vi "英维克空调.vi"() -> ()   [LabVIEW 2016, in "环境动力监测库.lvlib" / "空调库.lvlib"]
panel:
  out "x+1":u32
  in  "解除告警":bool
  out "串口":string
  in  "查看型号":bool
  out "遥控开关机状态":bool
  in  "重开串口":bool
  in  "设定参数":bool
  in  "遥控":bool
  out "系统参数":T1
  out "告警状态":T2
  out "传感器状态":T3
  out "运行状态":T4
  out "通讯":bool
  # "℃"
  # "℃"
  # "℃"
  # "℃"
  # "℃"
  # "℃"
  # "%"
  # "℃"
  # "℃"
  # "℃"
  # "℃"
  # "℃"
  # "%"
  # "℃"
  # "A"
  # "V"
  # "V"
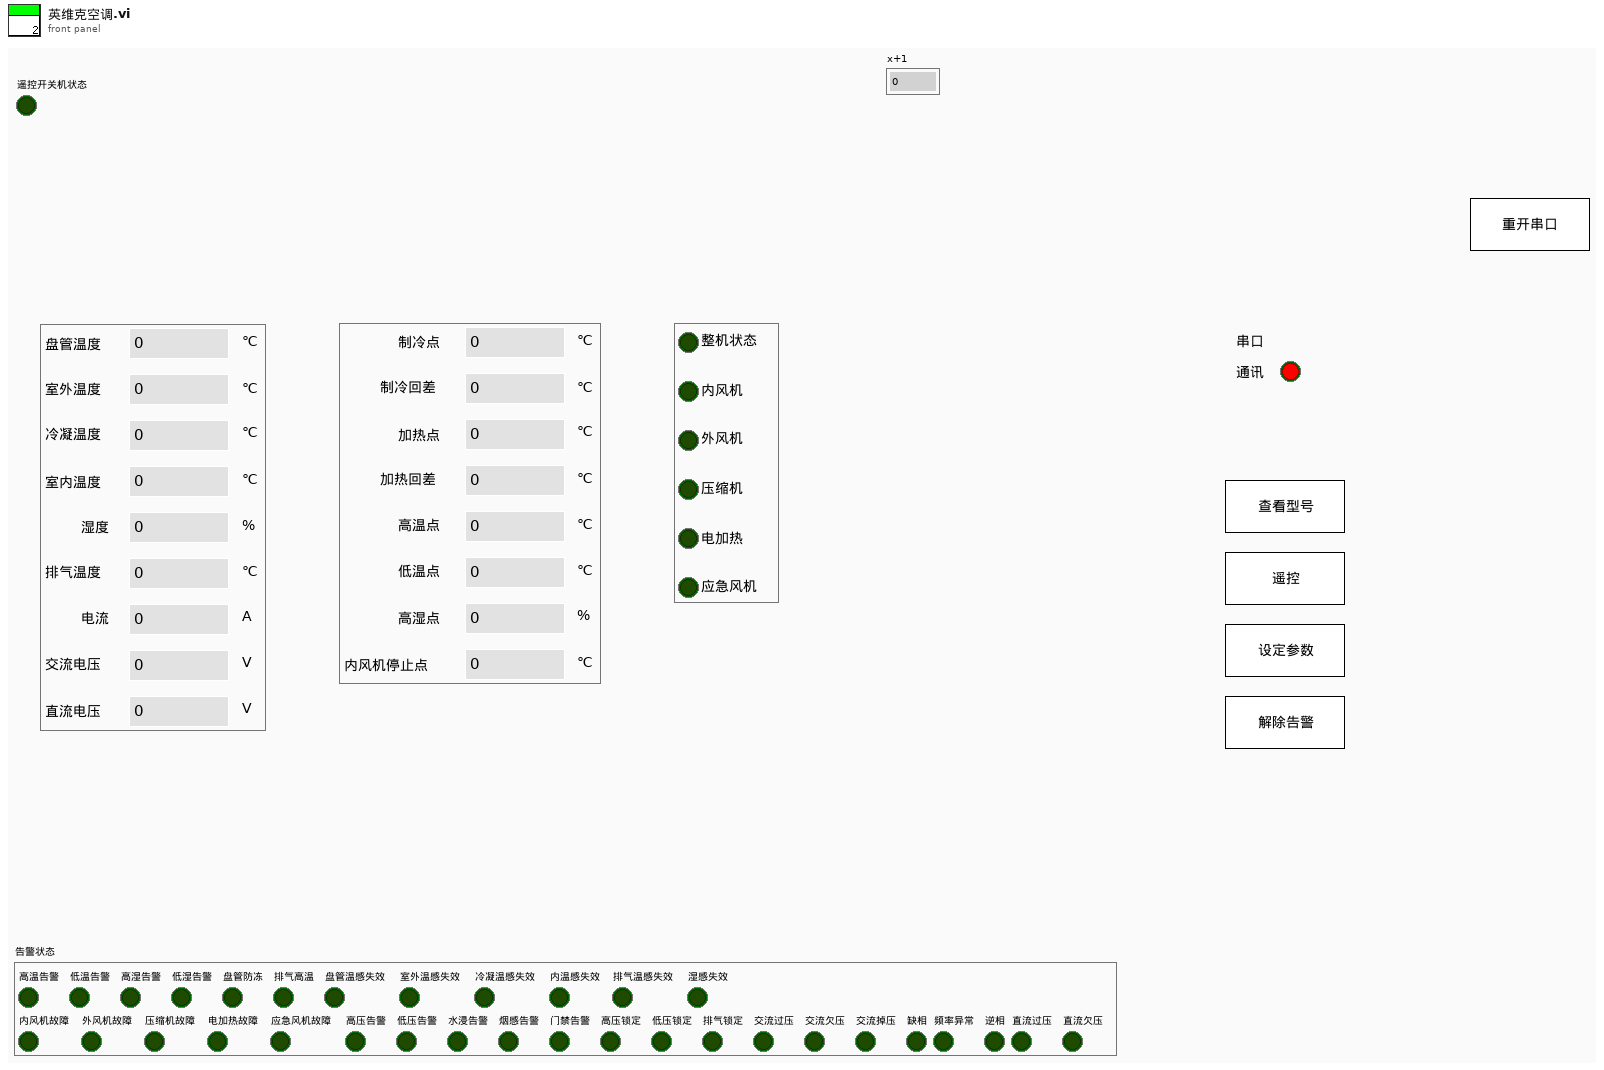
[diagram p1: front panel]
types:
  T1 = cluster{"制冷点":u16, "制冷回差":u16, "加热点":u16, "加热回差":u16, "预留":u16, "预留":u16, "高温点":u16, "低温点":u16, "高湿点":u16, "内风机停止点":u16}
  T2 = cluster{"高温告警":bool, "低温告警":bool, "高湿告警":bool, "低湿告警":bool, "盘管防冻":bool, "排气高温":bool, "盘管温感失效":bool, "室外温感失效":bool, "冷凝温感失效":bool, "内温感失效":bool, "排气温感失效":bool, "湿感失效":bool, "内风机故障":bool, "外风机故障":bool, "压缩机故障":bool, "电加热故障":bool, "应急风机故障":bool, "高压告警":bool, "低压告警":bool, "水浸告警":bool, "烟感告警":bool, "门禁告警":bool, "高压锁定":bool, "低压锁定":bool, "排气锁定":bool, "交流过压":bool, "交流欠压":bool, "交流掉压":bool, "缺相":bool, "频率异常":bool, "逆相":bool, "直流过压":bool, "直流欠压":bool}
  T3 = cluster{"盘管温度":u16, "室外温度":u16, "冷凝温度":u16, "室内温度":u16, "湿度":u16, "排气温度":u16, "电流":u16, "交流电压":u16, "直流电压":u16}
  T4 = cluster{"整机状态":bool, "内风机":bool, "外风机":bool, "压缩机":bool, "电加热":bool, "应急风机":bool}
  T5 = cluster{"型号选择":enum16{"黑盾", "英维克", "仁科测控RS-KTC-N01"}, "MB session in":refnum<class "MB_Master.lvclass">, "英维克空调寄存器":u16[], "通讯状态":bool, "PORT":string, "IP":string, "Slave ID ":u8, "Serial Config":cluster{"baud rate (bps)":u32, "stop bits":u16, "parity":u16, "flow control":u16, "timeout":u32, "retries":i32}, "VISA Resource":refnum<visa-resource-name>, "MB通信方式选择":enum16{"串口", "TCP"}, "系统参数":cluster{"空调开启点":u16, "空调灵敏点":u16, "加热开启点":u16, "加热灵敏度":u16, "高温告警点":u16, "低温告警点":u16}}
  T6 = cluster{"制冷点":u16, "制冷回差":u16, "加热点":u16, "加热回差":u16, "保留":u16, "保留":u16, "高温点":u16, "低温点":u16, "高湿点":u16, "内风机停止点":u16}
  T7 = cluster{"温湿度":cluster{"状态":bool, "温度:":sgl, "湿度:":sgl, "详情  ":bool}, "空调":cluster{"状态":bool, "机柜温度:":sgl, "压缩机:":enum16{"停止", "运行"}, "电加热:":enum16{"停止", "运行"}, "详情  ":bool}, "排气扇":cluster{"排气扇":bool, "详情  ":bool}, "冰箱":cluster{"冰箱":bool, "详情  ":bool}}
  T8 = enum16{"open", "read", "write single", "write", "close"}
  T9 = enum16{"空调制冷点", "空调制冷回差", "加热点", "加热回差", "高温点", "低温点", "高湿点", "内风机停止点"}
  T10 = cluster{"漏水监测输出":cluster{"漏水监测告警":bool, "告警内容":string}, "门禁监测输出":cluster{"门禁监测告警":bool, "告警内容":string}, "门禁监测输出2":cluster{"门禁监测告警":bool, "告警内容":string}, "温湿度监测输出":cluster{"温湿度监测告警":bool, "告警内容":string}, "烟雾监测输出":cluster{"烟雾监测告警":bool, "告警内容":string}, "空调监测输出":cluster{"空调监测告警":bool, "告警内容":string}, "自动重合闸输出":cluster{"自动重合闸告警":bool, "告警内容":string}, "红外入侵输出":cluster{"红外入侵告警":bool, "告警内容":string}, "振动输出":cluster{"振动告警":bool, "告警内容":string}, "UPS输出":cluster{"UPS告警":bool, "告警内容":string}, "蓄电池输出":cluster{"蓄电池告警":bool, "告警内容":string}, "蓄电池输出2":cluster{"蓄电池告警":bool, "告警内容":string}, "GPS输出":cluster{"定位告警":bool, "告警内容":string}, "北斗输出":cluster{"定位告警":bool, "告警内容":string}, "气象输出":cluster{"气象告警":bool, "告警内容":string}, "废液输出":cluster{"废液告警":bool, "告警内容":string}, "废液输出2":cluster{"废液告警":bool, "告警内容":string}}
  T11 = enum32{"Bad", "Idle", "Run top level", "Running"}
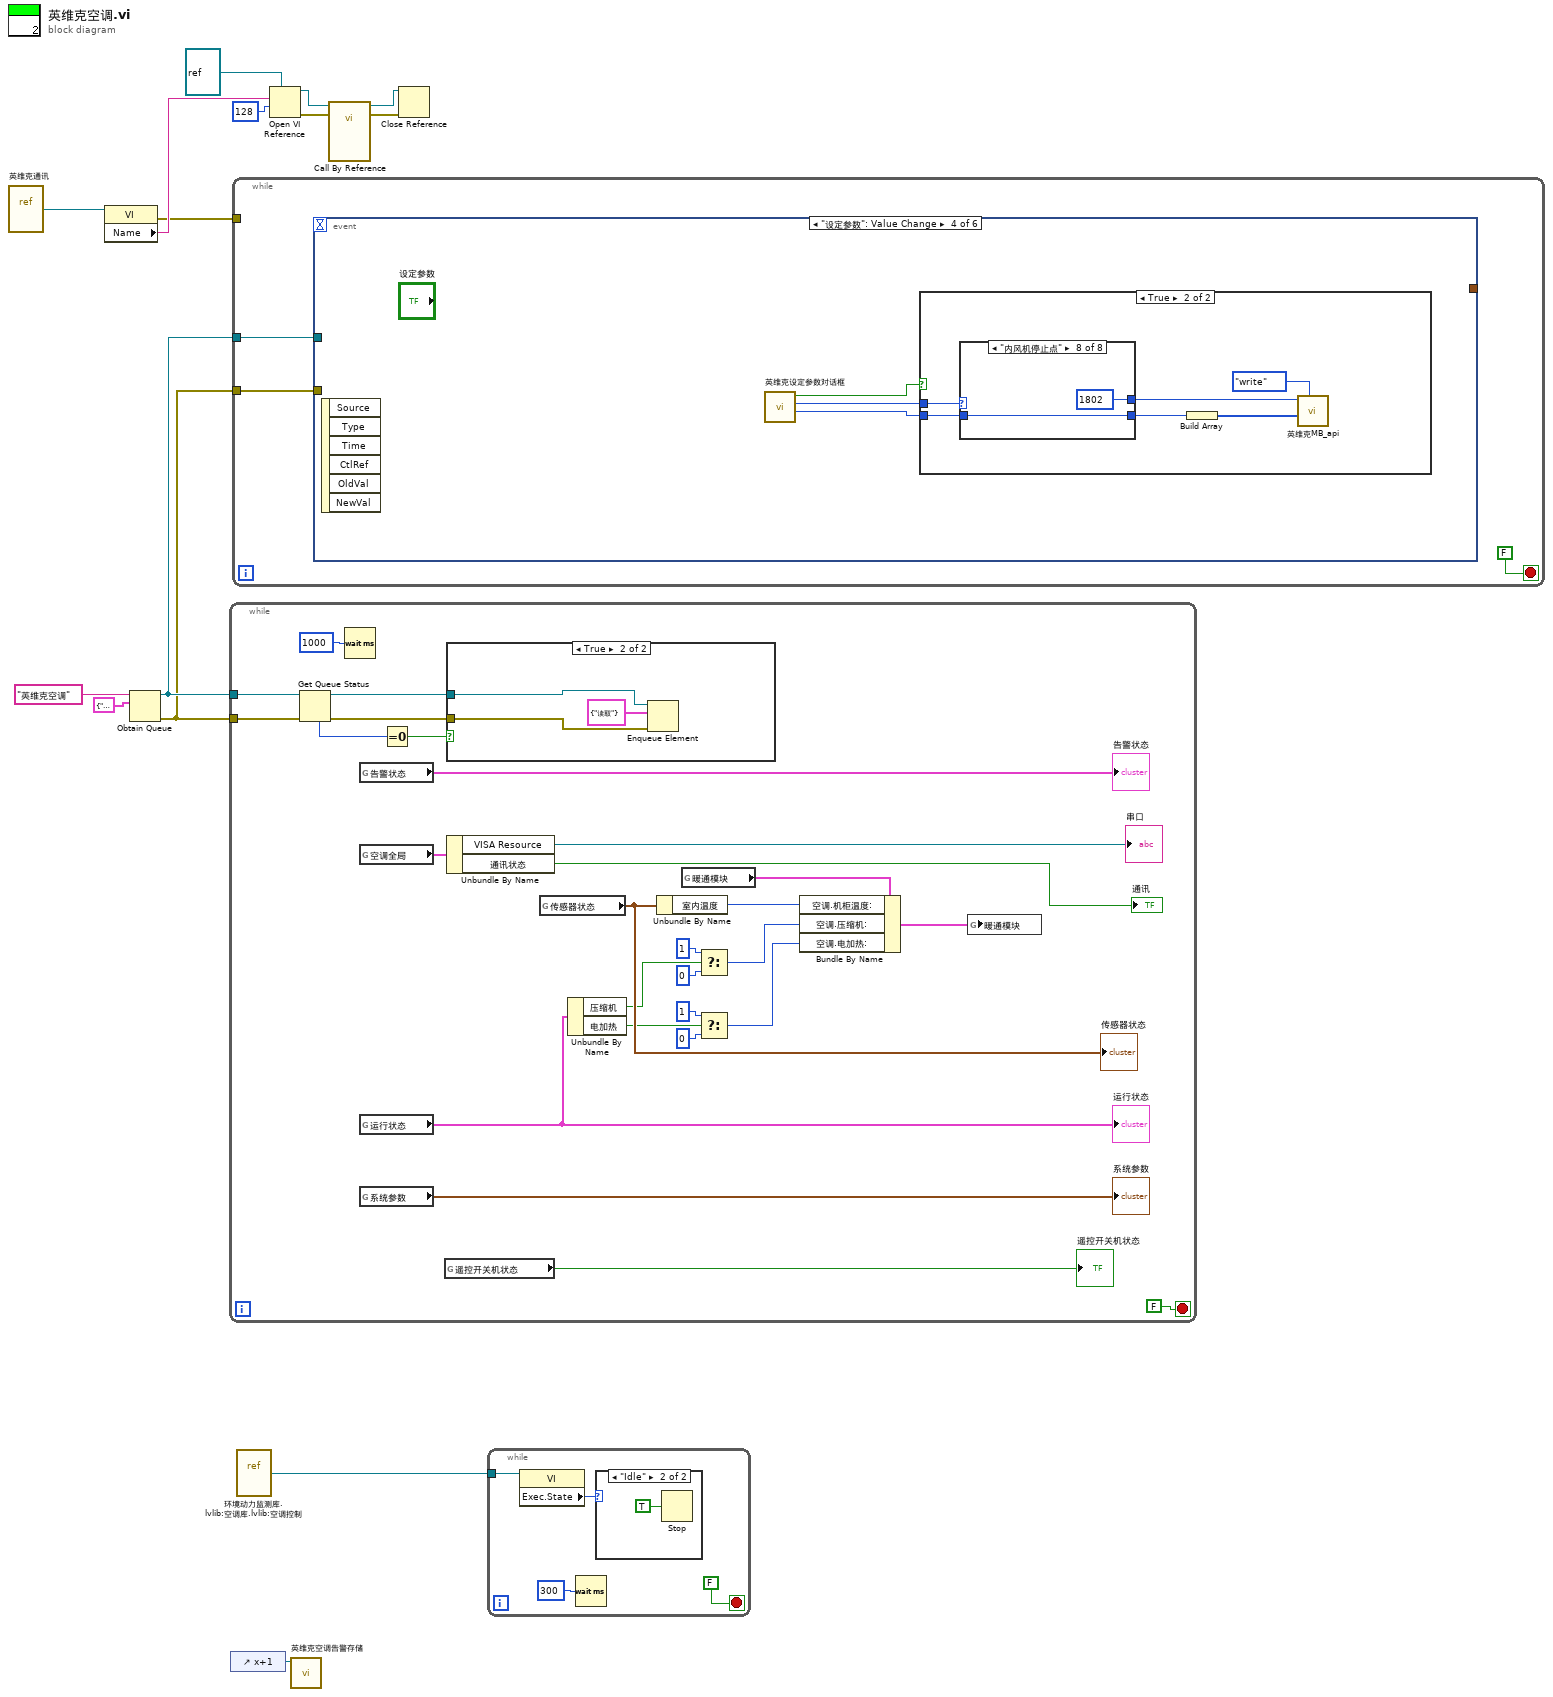
[diagram p0: block diagram]
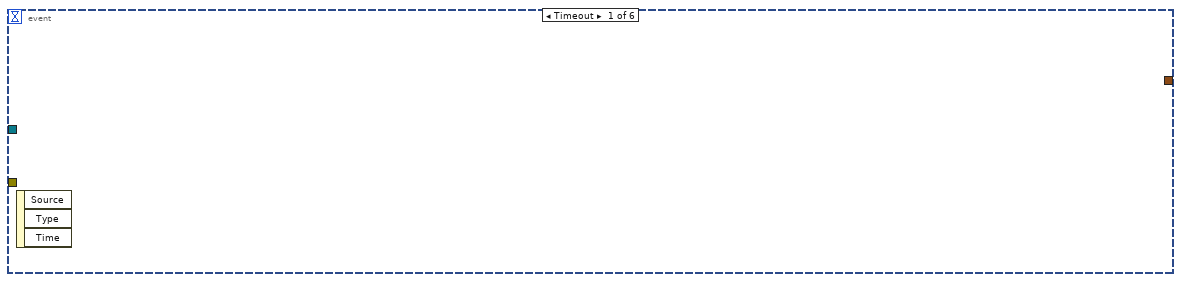
[diagram p4: hidden frame]
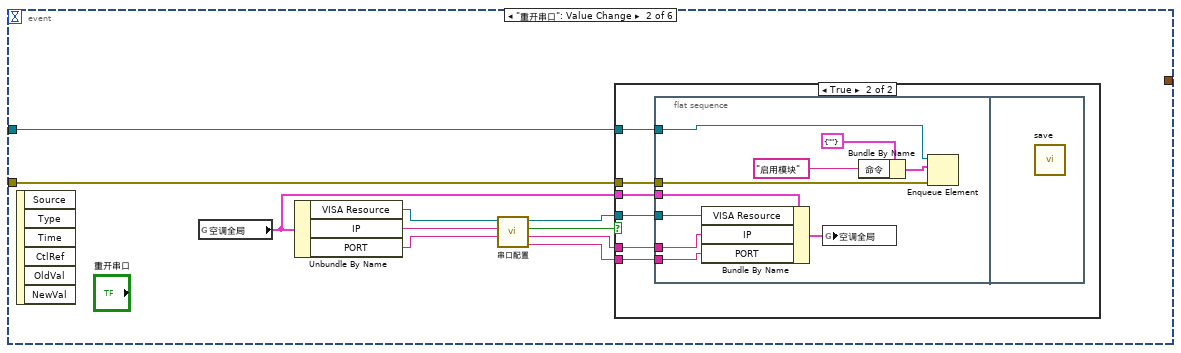
[diagram p5: hidden frame]
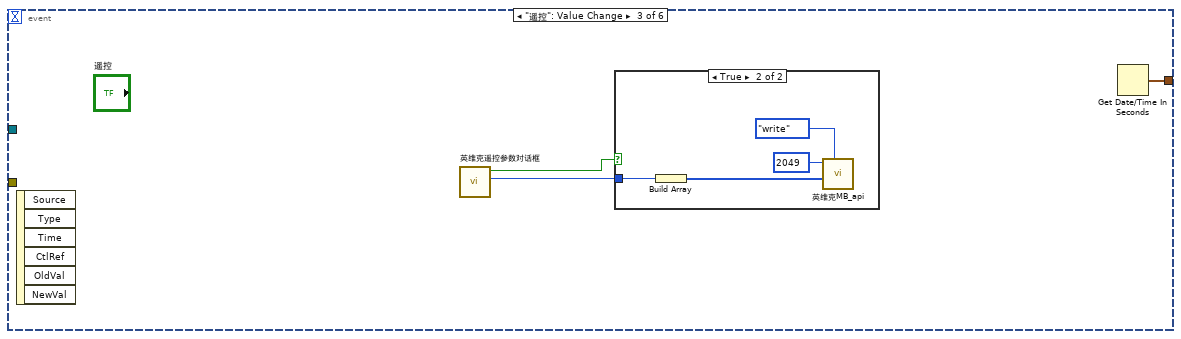
[diagram p7: hidden frame]
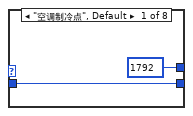
[diagram p10: hidden frame]
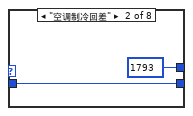
[diagram p11: hidden frame]
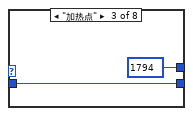
[diagram p12: hidden frame]
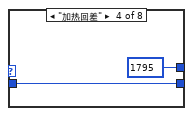
[diagram p13: hidden frame]
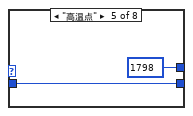
[diagram p14: hidden frame]
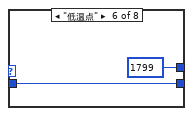
[diagram p15: hidden frame]
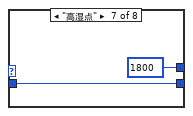
[diagram p16: hidden frame]
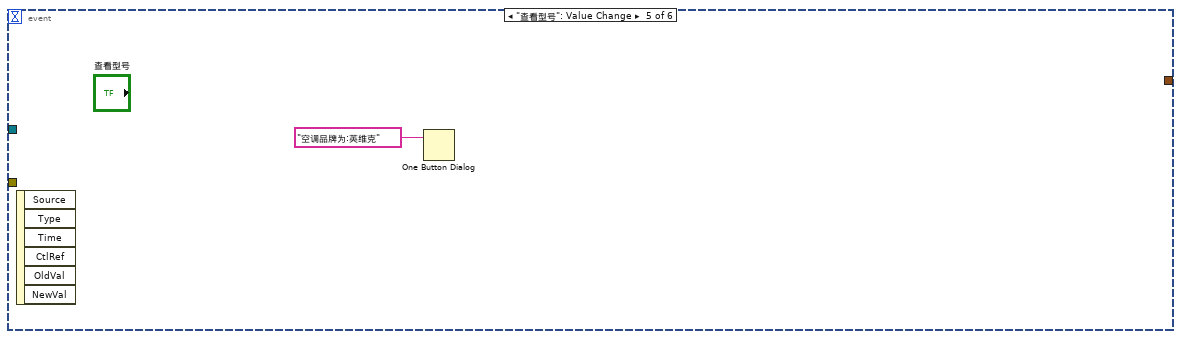
[diagram p17: hidden frame]
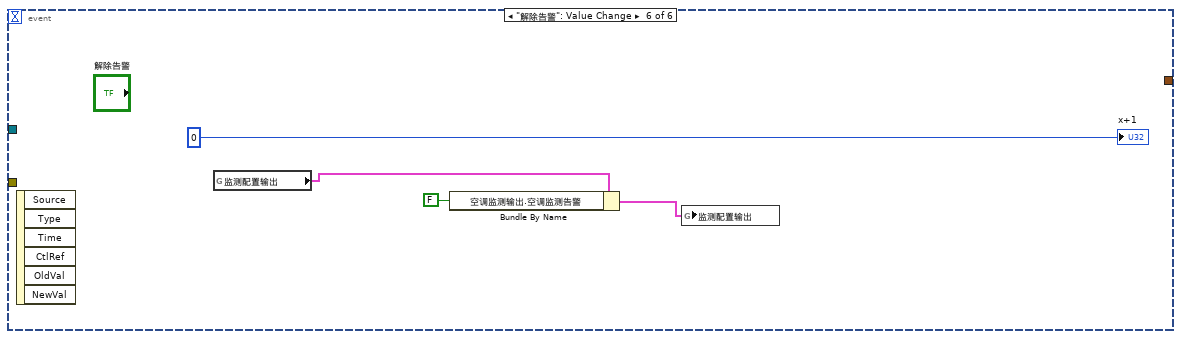
[diagram p18: hidden frame]
diagram:
  n1 = vi-ref "英维克通讯.vi"() -> (w8:refnum<vi>)
  n2 = property class="VI"(reference=w8) -> (error out=w3:errorcluster, "Name"=w9:string)  [unwired: 1 in, 1 out]
  n3 = Obtain Queue(name (unnamed)="英维克空调" ("名称（未命名）"), element data type=cluster{"命令":string} {"命令"="启用模块"} ("元素")) -> (queue out=w5:refnum<queue>, error out=w4:errorcluster)  [unwired: 3 in, 1 out]
  n4 = while {
    tunnel: w5 -> [w41]
    tunnel: w4 -> [w40]
    stop <- FALSE stop-if-true
    n5 = Get Queue Status(queue=w41, error in (no error)=w40) -> (queue out=w38:refnum<queue>, error out=w37:errorcluster, # elements in queue=w42:i32)  [unwired: 1 in, 5 out]
    n6 = Wait (ms)(milliseconds to wait=u32 1000 ("等待时间（毫秒）")) -> ()  [unwired: 1 out]
    n7 = global read "内部交互全局变量.vi" "告警状态"() -> (→"告警状态":T2)
    n8 = global read "断电保存全局变量.vi" "空调全局"() -> (w18:T5)
    n9 = global read "内部交互全局变量.vi" "运行状态"() -> (w27:T4)
    "运行状态" <- w27
    n10 = global read "内部交互全局变量.vi" "系统参数"() -> (→"系统参数":T6)
    n11 = Equal To 0?(x=w42) -> (x = 0?=w39:bool)
    n12 = global read "内部交互全局变量.vi" "遥控开关机状态"() -> (→"遥控开关机状态":bool)
    n13 = case shown="True" w39 {
      tunnel: w38 -> [_ w45]
      tunnel: w37 -> [_ w44]
      frame False {
      }
      frame True {
        n14 = Enqueue Element(queue=w45, element=cluster{"命令":string} {"命令"="读取"} ("元素"), error in (no error)=w44) -> ()  [unwired: 1 in, 3 out]
      }
    }
    n15 = Unbundle By Name(w18) -> ("VISA Resource"=→"串口":refnum<visa-resource-name>, "通讯状态"=→"通讯":bool)
    n16 = global read "内部交互全局变量.vi" "传感器状态"() -> (w29:T3)
    "传感器状态" <- w29
    n17 = Unbundle By Name(w27) -> ("压缩机"=w26:bool, "电加热"=w21:bool)
    n18 = Unbundle By Name(w29) -> ("室内温度"=w28:u16)
    n19 = global read "内部交互全局变量.vi" "暖通模块"() -> (w30:T7)
    n20 = Select(t=1, s=w26, f=0) -> (s? t:f=w20:i32)
    n21 = Select(t=1, s=w21, f=0) -> (s? t:f=w19:i32)
    n22 = Bundle By Name(cluster=w30, "空调.机柜温度:"=w28, "空调.压缩机:"=w20, "空调.电加热:"=w19) -> (w31:T7)
    n23 = global write "内部交互全局变量.vi" "暖通模块"(w31) -> ()
  }
  n24 = control-ref of="x+1"() -> (w1:refnum<vi>)
  n25 = while {
    tunnel: w5 -> [w47]
    tunnel: w4 -> [w46]
    tunnel: w3 -> [_]
    stop <- FALSE stop-if-true
    n26 = event shown="[3] \"设定参数\": Value Change" {
      selector: _ -> [_ _ _ _ _ _]
      dyn-events: _ -> [_ _ _ _ _ _]
      timeout: _ -> [_ _ _ _ _ _]
      tunnel: w47 -> [_ w54 _ _ _ _]
      tunnel: w46 -> [_ w53 _ _ _ _]
      tunnel: [_ _ w75 _ _ _] -> _
      event Timeout {
        n27 = event-data() -> ()  [unwired: 1 in, 3 out]
      }
      event "重开串口": Value Change {
        n28 = event-data() -> ()  [unwired: 1 in, 6 out]
        n29 = global read "断电保存全局变量.vi" "空调全局"() -> (w49:T5)
        n30 = Unbundle By Name(w49) -> ("VISA Resource"=w52:refnum<visa-resource-name>, "IP"=w51:string, "PORT"=w50:string)
        n31 = call "串口配置.vi"("PORT"=w50, "IP"=w51, "请选择串口:"=w52) -> ("PORT 2"=w55:string, "IP 2"=w56:string, "确认 2"=w57:bool, "VISA资源名称 2"=w58:refnum<visa-resource-name>)  [unwired: 5 in]
        n32 = case shown="True" w57 {
          tunnel: w58 -> [_ w62]
          tunnel: w54 -> [_ w64]
          tunnel: w53 -> [_ w63]
          tunnel: w56 -> [_ w61]
          tunnel: w55 -> [_ w60]
          tunnel: w49 -> [_ w59]
          frame False {
          }
          frame True {
            n33 = flat-sequence {
              tunnel: w64 -> [w71]
              tunnel: w63 -> [w70]
              tunnel: w62 -> [w67]
              tunnel: w61 -> [w66]
              tunnel: w60 -> [w65]
              tunnel: w59 -> [w69]
              frame #0 {
                n34 = Bundle By Name(cluster=w69, "VISA Resource"=w67, "IP"=w66, "PORT"=w65) -> (w68:T5)
                n35 = global write "断电保存全局变量.vi" "空调全局"(w68) -> ()
                n36 = Bundle By Name(cluster=cluster{"命令":string} {"命令"=""} ("元素"), "命令"="启用模块" ("名称（未命名）")) -> (w72:cluster{"命令":string})
                n37 = Enqueue Element(queue=w71, element=w72, error in (no error)=w70) -> ()  [unwired: 1 in, 3 out]
              }
              frame #1 {
                n38 = call "save.vi"() -> ()  [unwired: 11 in, 1 out]
              }
            }
          }
        }
      }
      event "遥控": Value Change {
        n39 = event-data() -> ()  [unwired: 1 in, 6 out]
        n40 = call "英维克遥控参数对话框.vi"() -> ("遥控参数选择输出"=w76:enum16{"空调关机", "空调开机"}, "确定?"=w77:bool)  [unwired: 10 in]
        n41 = case shown="True" w77 {
          tunnel: w76 -> [_ w80]
          frame False {
          }
          frame True {
            n42 = Build Array(w80) -> (w79:enum16{"空调关机", "空调开机"}[])
            n43 = call "英维克MB_api.vi"("STEP"=T8."write", "values"=w79, "starting address"=u16 2049) -> ()  [unwired: 6 in, 3 out]
          }
        }
        n44 = Get Date/Time In Seconds() -> (seconds since 1Jan1904=w75:timestamp)
      }
      event "设定参数": Value Change {
        n45 = event-data() -> ()  [unwired: 1 in, 6 out]
        n46 = call "英维克设定参数对话框.vi"() -> ("参数 2"=w82:u16, "设定参数（定点数）选择 2"=w83:T9, "确定?"=w84:bool)  [unwired: 9 in]
        n47 = case shown="True" w84 {
          tunnel: w83 -> [_ w90]
          tunnel: w82 -> [_ w87]
          frame False {
          }
          frame True {
            n48 = case shown="\"内风机停止点\"" w90 {
              tunnel: [u16 1792 ("starting address") u16 1793 ("starting address") u16 1794 ("starting address") u16 1795 ("starting address") u16 1798 ("starting address") u16 1799 ("starting address") u16 1800 ("starting address") u16 1802 ("starting address")] -> w88
              tunnel: w87 -> [w91 w93 w95 w97 w99 w101 w103 w105]
              tunnel: [w91 w93 w95 w97 w99 w101 w103 w105] -> w86
              frame "空调制冷点", Default {
              }
              frame "空调制冷回差" {
              }
              frame "加热点" {
              }
              frame "加热回差" {
              }
              frame "高温点" {
              }
              frame "低温点" {
              }
              frame "高湿点" {
              }
              frame "内风机停止点" {
              }
            }
            n49 = Build Array(w86) -> (w89:u16[])
            n50 = call "英维克MB_api.vi"("STEP"=T8."write", "values"=w89, "starting address"=w88) -> ()  [unwired: 6 in, 3 out]
          }
        }
      }
      event "查看型号": Value Change {
        n51 = event-data() -> ()  [unwired: 1 in, 6 out]
        n52 = One Button Dialog(message="空调品牌为:英维克" ("消息")) -> ()  [unwired: 1 in, 1 out]
      }
      event "解除告警": Value Change {
        n53 = event-data() -> ()  [unwired: 1 in, 6 out]
        n54 = global read "内部交互全局变量.vi" "监测配置输出"() -> (w109:T10)
        n55 = Bundle By Name(cluster=w109, "空调监测输出.空调监测告警"=FALSE) -> (w108:T10)
        n56 = global write "内部交互全局变量.vi" "监测配置输出"(w108) -> ()
        "x+1" <- u32 0 ("x+1")
      }
    }
  }
  n57 = vi-ref "环境动力监测库.lvlib:空调库.lvlib:空调控制.vi"() -> (w2:refnum<vi>)
  n58 = Open VI Reference(type specifier VI Refnum (for type only)=refnum<vi> refnum, vi path=w9, options=128 ("选项")) -> (vi reference=w11:refnum<vi>, error out=w13:errorcluster)  [unwired: 3 in]
  n59 = call "英维克空调告警存储.vi"("x+1"=w1) -> ()  [unwired: 11 in]
  n60 = call-by-ref "?"(reference=w11, error in=w13) -> (reference out=w15:refnum<vi>, error out=w14:errorcluster)  [unwired: 12 in]
  n61 = Close Reference(reference=w15, error in (no error)=w14) -> ()  [unwired: 1 out]
  n62 = while {
    tunnel: w2 -> [w115]
    stop <- FALSE stop-if-true
    n63 = property class="VI"(reference=w115) -> ("Exec.State"=w114:T11)  [unwired: 1 in, 2 out]
    n64 = Wait (ms)(milliseconds to wait=u32 300 ("等待时间（毫秒）")) -> ()  [unwired: 1 out]
    n65 = case shown="\"Idle\"" w114 {
      frame "Bad", Default {
      }
      frame "Idle" {
        n66 = Stop(stop? (T)=TRUE ("停止？(T)")) -> ()
      }
    }
  }
